vi "Define Ramp Array Dialog.vi"(8 "error in (no error)":errorcluster) -> (0 "error out":errorcluster, 1 "OK?":bool caption="OK", 3 "Ramp":dbl[](array[numeric]))   [LabVIEW 2021, in "Arrays.lvlib"]
uses:
  Arrays.lvlib
  <vilib>/Analysis/1siggen.llb/Ramp Pattern by Samples.vi
  <vilib>/Analysis/1siggen.llb/Ramp Pattern by Delta.vi
  <vilib>/Analysis/NI_AALBase.lvlib
panel:
  in  "Delta":dbl caption="Start" format="%#g"
  in  "Exclude End?":bool
  in  "Spacing":enum16{"Linear", "Logarithmic"}(ring)
  in  "Ramp Type":enum16{"Ramp by Sample", "Ramp by Delta"}(ring)
  in  "End":dbl format="%#g"
  in  "Start":dbl format="%#g"
  in  "# Samples":i32=1 caption="Ramp Type" min=1
  in  "Cancel":bool
  in  "OK":bool caption="OK2"
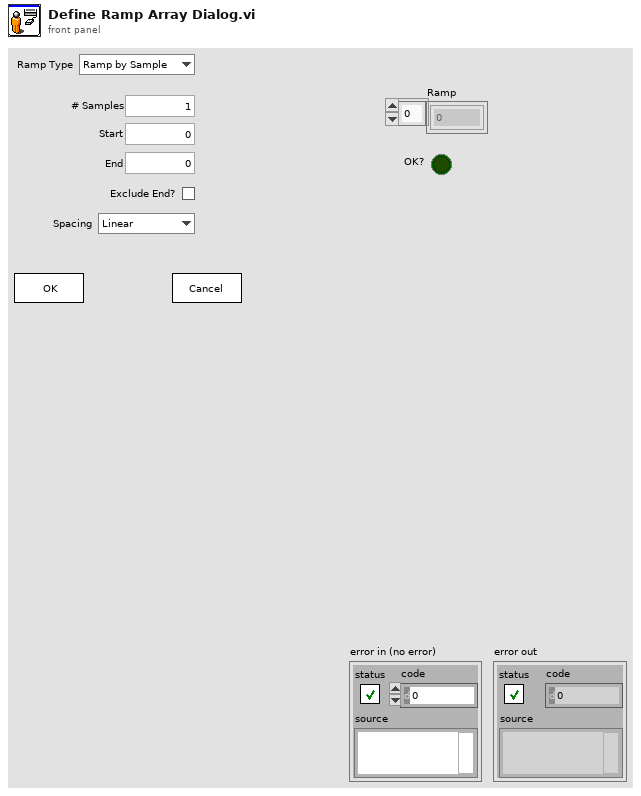
[diagram p1: front panel]
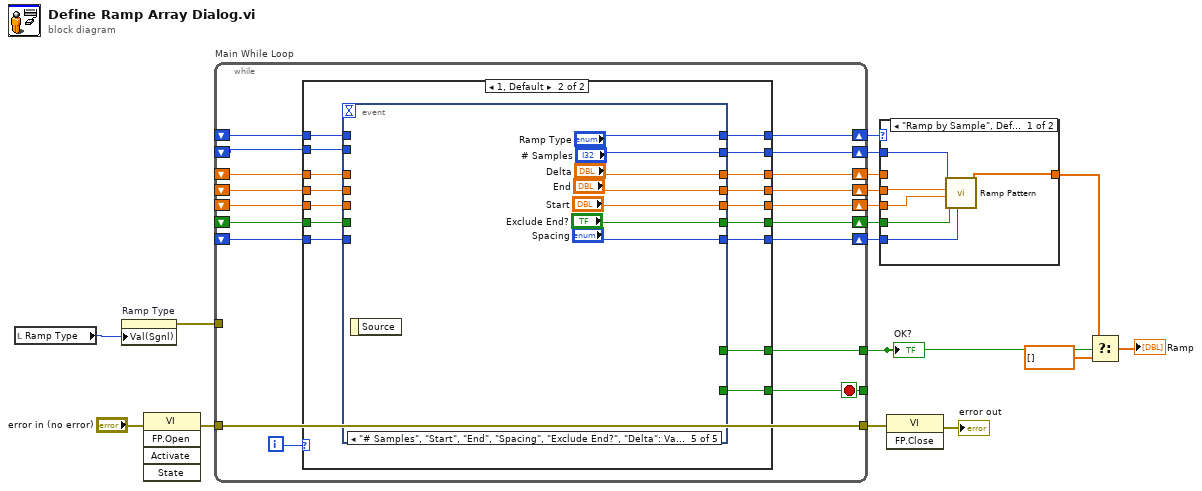
[diagram p0: block diagram]
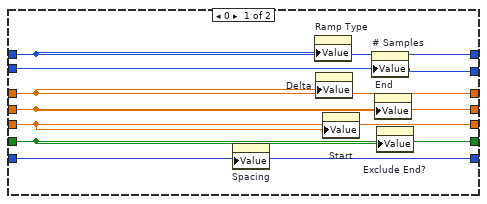
[diagram p2: hidden frame]
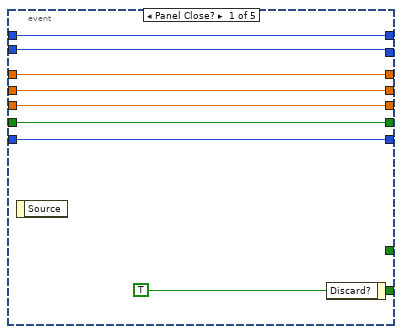
[diagram p3: hidden frame]
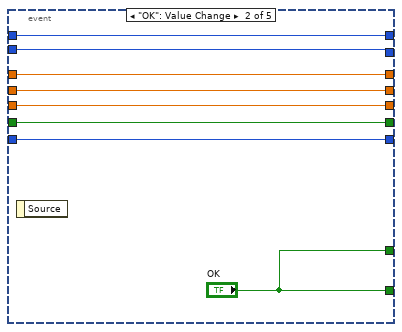
[diagram p4: hidden frame]
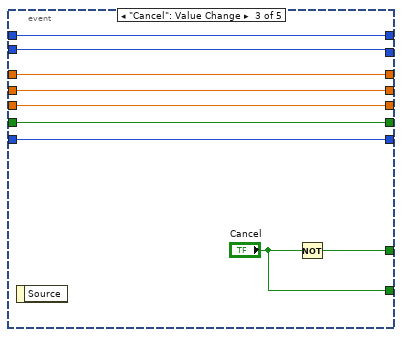
[diagram p5: hidden frame]
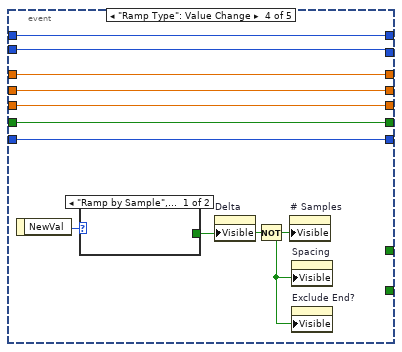
[diagram p6: hidden frame]
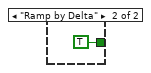
[diagram p7: hidden frame]
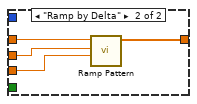
[diagram p8: hidden frame]
diagram:
  n1 = local read "Ramp Type"() -> (w2:enum16{"Ramp by Sample", "Ramp by Delta"})
  n2 = property on="Ramp Type" class="Enum (strict)"("Val(Sgnl)"=w2) -> (error out=w1:errorcluster)  [unwired: 2 in, 1 out]
  n3 = invoke class="VI" method="FP.Open"(error in="error in (no error)") -> (error out=w17:errorcluster)  [unwired: 4 in, 4 out]
  n4 = while "Main While Loop" {
    tunnel: w17 -> [w35]
    tunnel: [w35] -> w15
    tunnel: [w34] -> _
    tunnel: [w33] -> w6
    tunnel: w1 -> [_]
    shift-right: [w32] -> w13
    shift-left: _ -> [w24]
    shift-right: [w31] -> w9
    shift-left: _ -> [w23]
    shift-right: [w30] -> w12
    shift-left: _ -> [w22]
    shift-right: [w29] -> w10
    shift-left: _ -> [w21]
    shift-right: [w28] -> w11
    shift-left: _ -> [w20]
    shift-right: [w27] -> w8
    shift-left: _ -> [w19]
    shift-right: [w26] -> w7
    shift-left: _ -> [w18]
    i -> [w25]
    stop <- w34 stop-if-true
    n5 = case shown="1, Default" w25 {
      tunnel: [_ w58] -> w34
      tunnel: [_ w57] -> w33
      tunnel: [w42 w56] -> w32
      tunnel: [w41 w55] -> w31
      tunnel: [w40 w54] -> w30
      tunnel: [w39 w53] -> w29
      tunnel: [w38 w52] -> w28
      tunnel: [w37 w51] -> w27
      tunnel: [w36 w50] -> w26
      tunnel: w24 -> [w42 w49]
      tunnel: w23 -> [w41 w48]
      tunnel: w22 -> [w40 w47]
      tunnel: w21 -> [w39 w46]
      tunnel: w20 -> [w38 w45]
      tunnel: w19 -> [w37 w44]
      tunnel: w18 -> [w36 w43]
      frame 0 {
        n6 = property on="Spacing" class="Enum (strict)"("Value"=w36) -> ()  [unwired: 2 in, 2 out]
        n7 = property on="Ramp Type" class="Enum (strict)"("Value"=w42) -> ()  [unwired: 2 in, 2 out]
        n8 = property on="Delta" class="DigNum (strict)"("Value"=w40) -> ()  [unwired: 2 in, 2 out]
        n9 = property on="Start" class="DigNum (strict)"("Value"=w38) -> ()  [unwired: 2 in, 2 out]
        n10 = property on="# Samples" class="DigNum (strict)"("Value"=w41) -> ()  [unwired: 2 in, 2 out]
        n11 = property on="End" class="DigNum (strict)"("Value"=w39) -> ()  [unwired: 2 in, 2 out]
        n12 = property on="Exclude End?" class="Bool (strict)"("Value"=w37) -> ()  [unwired: 2 in, 2 out]
      }
      frame 1, Default {
        n13 = event shown="[4] \"# Samples\", \"Start\", \"End\", \"Spacing\", \"Exclude End?\", \"Delta\": Value Change" {
          selector: _ -> [_ _ _ _ _]
          dyn-events: _ -> [_ _ _ _ _]
          timeout: _ -> [_ _ _ _ _]
          tunnel: [w66 "OK" "Cancel" _ _] -> w58
          tunnel: [_ "OK" w82 _ _] -> w57
          tunnel: [w65 w73 w81 w90 "Ramp Type"] -> w56
          tunnel: [w64 w72 w80 w89 "# Samples"] -> w55
          tunnel: [w63 w71 w79 w88 "Delta"] -> w54
          tunnel: [w62 w70 w78 w87 "End"] -> w53
          tunnel: [w61 w69 w77 w86 "Start"] -> w52
          tunnel: [w60 w68 w76 w85 "Exclude End?"] -> w51
          tunnel: [w59 w67 w75 w84 "Spacing"] -> w50
          tunnel: w49 -> [w65 w73 w81 w90 _]
          tunnel: w48 -> [w64 w72 w80 w89 _]
          tunnel: w47 -> [w63 w71 w79 w88 _]
          tunnel: w46 -> [w62 w70 w78 w87 _]
          tunnel: w45 -> [w61 w69 w77 w86 _]
          tunnel: w44 -> [w60 w68 w76 w85 _]
          tunnel: w43 -> [w59 w67 w75 w84 _]
          event Panel Close? {
            w66 = TRUE ("Discard?")
            n14 = event-data() -> ()  [unwired: 1 in, 1 out]
            n15 = event-data("Discard?"=w66) -> ()  [unwired: 1 in, 1 out]
          }
          event "OK": Value Change {
            n16 = event-data() -> ()  [unwired: 1 in, 1 out]
          }
          event "Cancel": Value Change {
            n17 = event-data() -> ()  [unwired: 1 in, 1 out]
            n18 = Not(x="Cancel") -> (.not. x?=w82:bool)
          }
          event "Ramp Type": Value Change {
            n19 = event-data() -> ("NewVal"=w93:enum16{"Ramp by Sample", "Ramp by Delta"})  [unwired: 1 in]
            n20 = case shown="\"Ramp by Sample\", Default" w93 {
              tunnel: [_ TRUE ("Visible")] -> w92
              frame "Ramp by Sample", Default {
              }
              frame "Ramp by Delta" {
              }
            }
            n21 = property on="Delta" class="DigNum (strict)"("Visible"=w92) -> ()  [unwired: 2 in, 2 out]
            n22 = Not(x=w92) -> (.not. x?=w91:bool)
            n23 = property on="# Samples" class="DigNum (strict)"("Visible"=w91) -> ()  [unwired: 2 in, 2 out]
            n24 = property on="Spacing" class="Enum (strict)"("Visible"=w91) -> ()  [unwired: 2 in, 2 out]
            n25 = property on="Exclude End?" class="Bool (strict)"("Visible"=w91) -> ()  [unwired: 2 in, 2 out]
          }
          event "# Samples", "Start", "End", "Spacing", "Exclude End?", "Delta": Value Change {
            n26 = event-data() -> ()  [unwired: 1 in, 1 out]
          }
        }
      }
    }
  }
  "OK?" <- w6
  n27 = case shown="\"Ramp by Sample\", Default" w13 {
    tunnel: w12 -> [_ w111]
    tunnel: w11 -> [w105 w110]
    tunnel: w10 -> [w106 w109]
    tunnel: [w102 w108] -> w5
    tunnel: w9 -> [w107 _]
    tunnel: w8 -> [w104 _]
    tunnel: w7 -> [w103 _]
    frame "Ramp by Sample", Default {
      n28 = call-poly <vilib>:"Ramp Pattern.vi"("type"=w103, "exclude end?"=w104, "start"=w105, "end"=w106, "samples"=w107) -> ("Ramp Pattern"=w102:dbl[])  [unwired: 5 in, 1 out]
    }
    frame "Ramp by Delta" {
      n29 = call-poly <vilib>:"Ramp Pattern.vi"("start"=w110, "end"=w109, "delta"=w111) -> ("Ramp Pattern"=w108:dbl[])  [unwired: 6 in, 2 out]
    }
  }
  n30 = invoke class="VI" method="FP.Close"(error in=w15) -> (error out=→"error out":errorcluster)  [unwired: 2 in, 2 out]
  n31 = Select(t=w5, s=w6, f=dbl[] []) -> (s? t:f=→"Ramp":dbl[])
